vi "PH_Stepmotor_BaseClass.Axis DIM remove Services.vi"(0 "IDs":T1) -> ()   [LabVIEW 2014, in "PH_Stepmotor_BaseClass.lvlib"]
doc: "This VI removes several DIM services of a motion axis."
uses:
  PH_Stepmotor_BaseClass.lvlib
  PH_Stepmotor_BaseClass.Axis DIM Service IDs.ctl
  lib.lib/DimLVEvent/LVDimInterface/LVDimInterface.lvlib
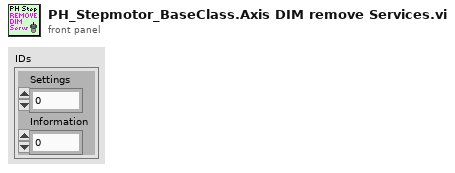
[diagram p1: front panel]
types:
  T1 = typedef "PH_Stepmotor_BaseClass.lvlib/PH_Stepmotor_BaseClass.Axis DIM Service IDs.ctl" = cluster{"Settings":i32, "Information":i32}
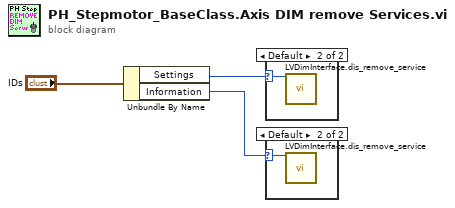
[diagram p0: block diagram]
diagram:
  n1 = Unbundle By Name("IDs") -> ("Settings"=w2:i32, "Information"=w3:i32)
  n2 = case shown="Default" w2 {
    selector: w2 -> [_ w4]
    frame -1 {
    }
    frame Default {
      n3 = call "LVDimInterface.dis_remove_service.vi"("my_serviceID"=w4) -> ()  [unwired: 18 in, 1 out]
    }
  }
  n4 = case shown="Default" w3 {
    selector: w3 -> [_ w5]
    frame -1 {
    }
    frame Default {
      n5 = call "LVDimInterface.dis_remove_service.vi"("my_serviceID"=w5) -> ()  [unwired: 18 in, 1 out]
    }
  }
